vi "test_launch-stopValidation.vi"(11 "Test Case In":refnum<class "TaskControllerTests.lvclass">) -> (0 "error out":errorcluster, 3 "Test Case Out":refnum<class "TaskControllerTests.lvclass">)   [LabVIEW 2023, in "TaskControllerTests.lvclass"]
uses:
  TaskControllerTests.lvclass
  <vilib>/Astemes/LUnit/Test Case.lvclass/Test Case.ctl
  <vilib>/Astemes/LUnit/Core/LUnit Test Case/Private/Append Fail Result.vi
  <vilib>/Astemes/LUnit/Core/LUnit Test Case/Private/Append Pass Result.vi
  <vilib>/Astemes/LUnit/Core/LUnit Test Case/Private/Run In UI.vi
  <vilib>/Utility/error.llb/Clear Errors.vi
  TLC_Connect/source/LabVIEW/TaskMock/TaskMock.lvclass
  TLC_Connect/source/LabVIEW/TaskController/TaskController.lvclass
  <vilib>/Astemes/LUnit/Test Case.lvclass
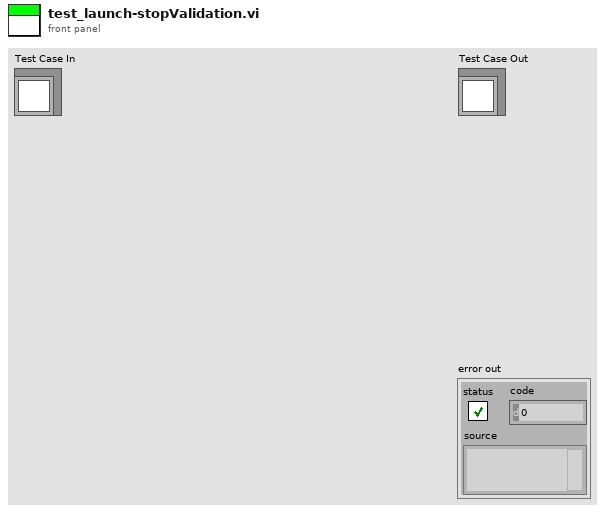
[diagram p1: front panel]
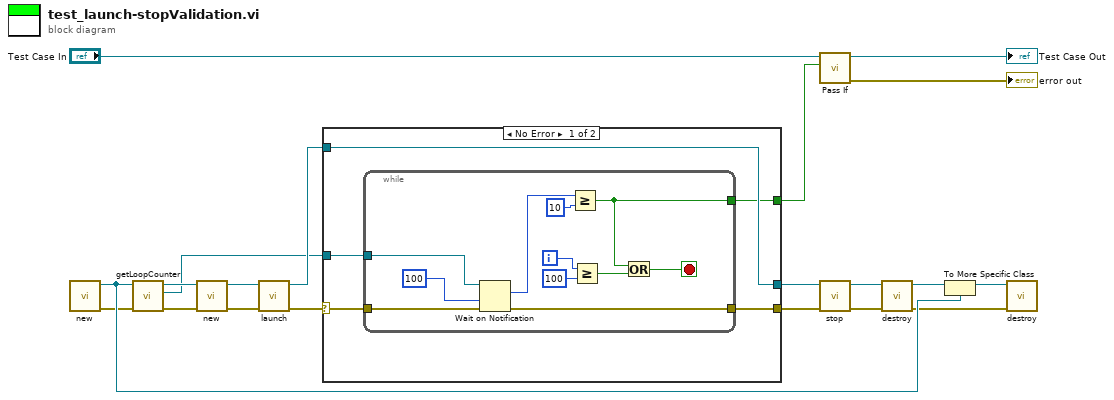
[diagram p0: block diagram]
diagram:
  n1 = call "new.vi"() -> ("error out"=w2:errorcluster, "TaskMock out"=w7:refnum<class "TaskMock.lvclass">)  [unwired: 10 in]
  n2 = call "getLoopCounter.vi"("error in (no error)"=w2, "TaskMock in"=w7) -> ("error out"=w1:errorcluster, "loopCounter"=w12:refnum<notifier>, "TaskMock out"=w13:refnum<class "TaskMock.lvclass">)  [unwired: 7 in]
  n3 = call "new.vi"("error in (no error)"=w1, "task"=w13) -> ("error out"=w16:errorcluster, "TaskController out"=w17:refnum<class "TaskController.lvclass">)  [unwired: 8 in]
  n4 = call "launch.vi"("error in (no error)"=w16, "TaskController in"=w17) -> ("error out"=w14:errorcluster, "TaskController out"=w15:refnum<class "TaskController.lvclass">)  [unwired: 8 in]
  n5 = case shown="No Error" w14 {
    selector: w14 -> [w25 _]
    tunnel: w15 -> [w23 w37]
    tunnel: w12 -> [w24 _]
    tunnel: [w23 w37] -> w11
    tunnel: [w22 _] -> w10
    tunnel: [w21 _] -> w3
    frame No Error {
      n6 = while {
        tunnel: w25 -> [w27]
        tunnel: w24 -> [w36]
        tunnel: [w30] -> w21
        tunnel: [w26] -> w22
        i -> [w32]
        stop <- w29 stop-if-true
        n7 = Wait on Notification(notifier=w36, timeout in ms (-1)=100, error in (no error)=w27) -> (notification=w34:i32, error out=w26:errorcluster)  [unwired: 1 in, 2 out]
        n8 = Greater Or Equal?(x=w34, y=10) -> (x >= y?=w30:bool)
        n9 = Greater Or Equal?(x=w32, y=100) -> (x >= y?=w28:bool)
        n10 = Or(x=w30, y=w28) -> (x .or. y?=w29:bool)
      }
    }
    frame Error {
    }
  }
  n11 = call <vilib>:"Pass If.vi"("Pass?"=w3, "LUnit Test Case In"="Test Case In") -> ("error out"=→"error out":errorcluster, "LUnit Test Case Out"=→"Test Case Out":refnum<class "TaskControllerTests.lvclass">)  [unwired: 8 in]
  n12 = call "stop.vi"("error in (no error)"=w10, "TaskController in"=w11) -> ("error out"=w8:errorcluster, "TaskController out"=w9:refnum<class "TaskController.lvclass">)  [unwired: 8 in]
  n13 = call "destroy.vi"("error in (no error)"=w8, "TaskController in"=w9) -> ("error out"=w6:errorcluster, "task"=w5:refnum<class "ITask.lvclass">)  [unwired: 8 in]
  n14 = To More Specific Class(target class=w7, reference=w5) -> (specific class reference=w4:refnum<class "TaskMock.lvclass">)  [unwired: 1 in, 1 out]
  n15 = call "destroy.vi"("error in (no error)"=w6, "TaskMock in"=w4) -> ()  [unwired: 9 in, 1 out]
